vi "Add Tab Button - Position Offset--Const.vi"() -> (3 "Position Offset":i32)   [LabVIEW 2017, in "DTacq Plot Display Library.lvlib"]
uses:
  DTacq Plot Display Library.lvlib
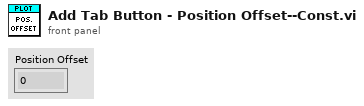
[diagram p1: front panel]
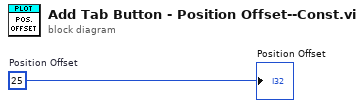
[diagram p0: block diagram]
diagram:
  w1 = 25  # Position Offset
  "Position Offset" <- w1
